vi "slink read energy w termination chars.vi"(8 "error in (no error)":errorcluster, 10 "# channels":i32, 11 "VISA Refnum in":refnum<visa-resource-name>) -> (0 "error out":errorcluster, 1 "Channel 2 value":dbl, 2 "Channel 1 value":dbl, 3 "VISA Refnum out":refnum<visa-resource-name>, 4 "AcqOkCh2":bool, 5 "String":string, 6 "AcqOkCh1":bool)   [LabVIEW 2020]
uses:
  Gentec Slink.lvclass
panel:
  out "Loop Time":u32
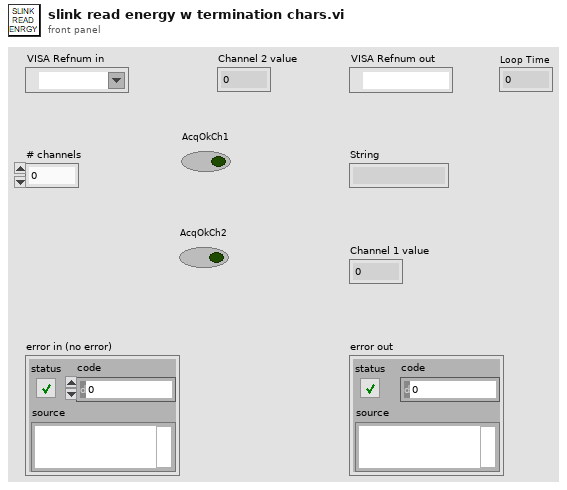
[diagram p1: front panel]
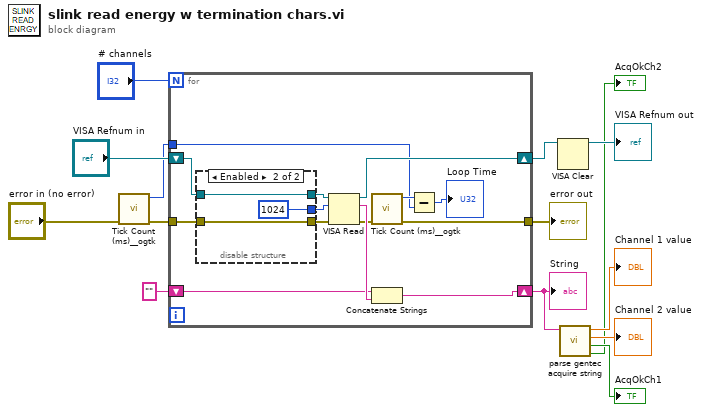
[diagram p0: block diagram]
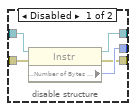
[diagram p2: hidden frame]
diagram:
  n1 = call "Tick Count (ms)__ogtk.vi"("error in (no error)"="error in (no error)") -> ("error out"=w2:errorcluster, "millisecond timer value"=w1:u32)  [unwired: 9 in]
  n2 = for {
    N: "# channels" -> [_]
    tunnel: [w18] -> w7
    shift-right: [w25] -> w13
    shift-left: "VISA Refnum in" -> [w24]
    shift-right: [w27] -> w8
    shift-left: "" -> [w26]
    tunnel: w2 -> [w21]
    tunnel: w1 -> [w16]
    n3 = disable-structure shown="Enabled" {
      disable-tunnel: w24 -> [w33 w36]
      disable-tunnel: [w32 w36] -> w23
      disable-tunnel: [w31 u32 1024 ("Bytes at Port")] -> w22
      disable-tunnel: w21 -> [w30 w35]
      disable-tunnel: [w29 w35] -> w20
      frame Disabled {
        n4 = property class="Instr"(reference=w33, error in=w30) -> (reference out=w32:refnum<visa-resource-name>, error out=w29:errorcluster, "Serial Settings:Number of Bytes at Serial Port"=w31:u32)
      }
      frame Enabled {
      }
    }
    n5 = VISA Read(VISA resource name=w23, byte count=w22, error in (no error)=w20) -> (VISA resource name out=w25:refnum<visa-resource-name>, read buffer=w28:string, error out=w19:errorcluster)  [unwired: 1 out]
    n6 = call "Tick Count (ms)__ogtk.vi"("error in (no error)"=w19) -> ("error out"=w18:errorcluster, "millisecond timer value"=w17:u32)  [unwired: 9 in]
    n7 = Concatenate Strings(w26, w28) -> (w27:string)
    n8 = Subtract(x=w17, y=w16) -> (x-y=→"Loop Time":u32)
  }
  "String" <- w8
  "error out" <- w7
  n9 = VISA Clear(VISA resource name=w13) -> (VISA resource name out=→"VISA Refnum out":refnum<visa-resource-name>)  [unwired: 1 in, 1 out]
  n10 = call "parse gentec acquire string.vi"("Acquisition String"=w8) -> ("AcqOkCh2"=→"AcqOkCh2":bool, "AcqOkCh1"=→"AcqOkCh1":bool, "Channel 2 value"=→"Channel 2 value":dbl, "Channel 1 value"=→"Channel 1 value":dbl)  [unwired: 7 in]
